vi "Clear Task.vi"(8 "error in":errorcluster, 11 "NI Analog Input in":refnum<class "NI Analog Input.lvclass">) -> (0 "error out":errorcluster, 3 "NI Analog Input out":refnum<class "NI Analog Input.lvclass">)   [LabVIEW 2023, in "HardwareAbstractionLayer_LVOOP.lvlib" / "NI Analog Input.lvclass"]
doc: "This VI DAXmx Clear Task"
uses:
  NI Analog Input.lvclass
  NI Analog Input.lvclass/NI Analog Input.ctl
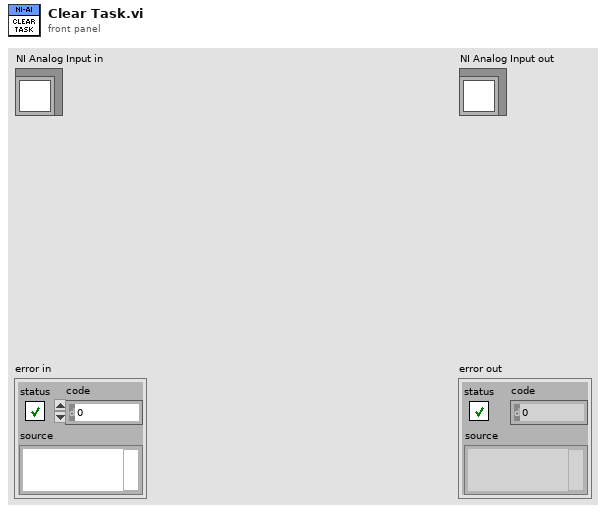
[diagram p1: front panel]
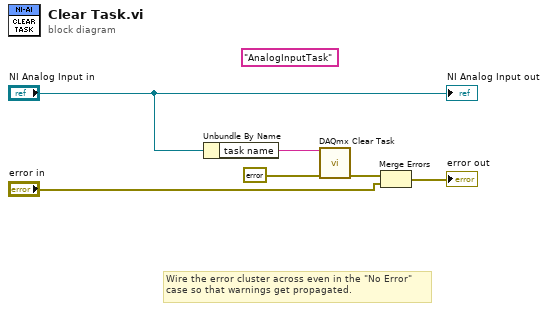
[diagram p0: block diagram]
diagram:
  (unwired) "AnalogInputTask" ("new task name")
  # "Wire the error cluster across even in the \"No Error\"\ncase so that warnings get propagated."
  n1 = Unbundle By Name("NI Analog Input in") -> ("task name"=w4:string)
  n2 = call <vilib>:"DAQmx Clear Task.vi"("task in"=w4, "error in"=errorcluster {"status"=FALSE, "code"=0, "source"=""}) -> ("error out"=w6:errorcluster)  [unwired: 13 in]
  n3 = Merge Errors(w6, "error in") -> (→"error out":errorcluster)
  "NI Analog Input out" <- "NI Analog Input in"
